vi "S4GUI_002.vi"(7 "Tab ObsEng":enum32{"Obs", "CCD modes", "Eng"}(tab)) -> ()   [LabVIEW 2018] (continued)
                    n514 = Number To Decimal String(number=w1082) -> (decimal integer string=w1084:string)  [unwired: 1 in]
                    n515 = Concatenate Strings("Disk Storage ", w1084, "%" ("string")) -> (w1081:string)
                    n516 = property on="Disk Storage ch3" class="Slide (strict)"("Caption.Text"=w1081) -> ()  [unwired: 2 in, 2 out]
                  }
                  frame #6 {
                    w1110 = cluster{u32, u32}[] [{16711680, 16711680}, {15400704, 15400704}, {16776722, 0}, {16776722, 0}]  # amarelo
                    w1109 = cluster{u32, u32}[] [{16711680, 16711680}, {6618880, 6618880}, {16776722, 0}, {16776722, 0}]  # verde
                    # "Se ocupacao do disco maior que\n90%, barra em vermelho."
                    # "Atualiza status CANAL4"
                    n517 = Unbundle By Name(w1122) -> ("Frames done"=w1117:u32, "connection"=→"Channel 4" →"setupCH4":bool, "conf runing"=w1121:bool, "UsedDisk"=w1103:u16, "operational"=w1107:bool)
                    "Exposures Done ch4" <- w1117
                    "Disk Storage ch4" <- w1103
                    n518 = Number To Decimal String(number=w1117) -> (decimal integer string=w1118:string)  [unwired: 1 in]
                    n519 = Greater?(x=w1103, y=u16 90) -> (0:w1114:bool)
                    n520 = Select(t=u32 16711680, s=w1114, f=u32 16860) -> (s? t:f=w1111:u32)
                    n521 = Concatenate Strings("#Exposures Done ", w1118) -> (w1116:string)
                    n522 = property on="setupCH4" class="Bool (strict)"("Blinking"=w1121) -> ()  [unwired: 2 in, 2 out]
                    n523 = property on="Disk Storage ch4" class="Slide (strict)"("Fill Color"=w1111) -> ()  [unwired: 2 in, 2 out]
                    n524 = Select(t=w1109, s=w1107, f=w1110) -> (s? t:f=w1108:cluster{u32, u32}[])
                    n525 = property on="Exposures Done ch4" class="Slide (strict)"("Caption.Text"=w1116) -> ()  [unwired: 2 in, 2 out]
                    n526 = property on="Channel 4" class="Bool (strict)"("Colors [4]"=w1108) -> ()  [unwired: 2 in, 2 out]
                    n527 = Number To Decimal String(number=w1103) -> (decimal integer string=w1105:string)  [unwired: 1 in]
                    n528 = Concatenate Strings("Disk Storage ", w1105, "%" ("string")) -> (w1102:string)
                    n529 = property on="Disk Storage ch4" class="Slide (strict)"("Caption.Text"=w1102) -> ()  [unwired: 2 in, 2 out]
                  }
                }
              }
              frame #9 {
                n530 = Unbundle By Name(w1128) -> ("Instrument Status.mode"=w1127:bool)
                n531 = case shown="True" w1127 {
                  tunnel: [0 ("t") w1141] -> w1124
                  tunnel: w1128 -> [_ w1130]
                  frame False {
                    # "Fotometria: #PSD = 0"
                  }
                  frame True {
                    # "Polarimetria: calcula #PSD"
                    n532 = Unbundle By Name(w1130) -> ("WPROT seq"=w1134:u16)
                    n533 = Number To Boolean Array(number=w1134) -> (Boolean array=w1133:bool[])
                    n534 = for {
                      shift-right: [w1145] -> w1136
                      shift-left: 0 -> [w1143]
                      tunnel: w1133 -> [w1142] mode=indexing
                      # "calcula qtd de 1s"
                      n535 = Increment(x=w1143) -> (x+1=w1144:i32)
                      n536 = Select(t=w1144, s=w1142, f=w1143) -> (s? t:f=w1145:i32)
                    }
                    n537 = property on="#Pol. Seq. Done" class="Slide (strict)"() -> ("Scale.Maximum"=w1135:dbl)  [unwired: 2 in, 2 out]
                    n538 = To Long Integer(number=w1135) -> (32bit integer=w1137:i32)
                    n539 = Subtract(x=w1137, y=w1136) -> (x-y=w1138:i32)
                    n540 = Decrement(x=w1138) -> (x-1=w1140:i32)
                    n541 = Less Than 0?(x=w1140) -> (x < 0?=w1139:bool)
                    n542 = Select(t=0, s=w1139, f=w1140) -> (s? t:f=w1141:i32)
                  }
                }
                "#Pol. Seq. Done" <- w1124
                n543 = Number To Decimal String(number=w1124) -> (decimal integer string=w1125:string)  [unwired: 1 in]
                n544 = Concatenate Strings("#Pol. Seq. Done ", w1125) -> (w1123:string)
                n545 = property on="#Pol. Seq. Done" class="Slide (strict)"("Caption.Text"=w1123) -> ()  [unwired: 2 in, 2 out]
              }
              frame #10 {
                # "OVJ 2022-12-12: \nA visibilidade do Tab ObsEng sempre \nacompanha a habilitação do tab4."
                n546 = Unbundle By Name(w1155) -> ("Cluster ExpMode.tab4"=w1149:T12, "Cluster Polarimetry"=w1176:T23, "Cluster Mode Sync"=w1183:T24)
                n547 = case shown="\"Enabled\", Default" w1149 {
                  tunnel: [TRUE ("Tabs Visible?") w1185] -> w1154
                  frame "Enabled", Default {
                  }
                  frame "Disabled and Grayed Out" {
                    n548 = disable-structure shown="Enabled" {
                      disable-tunnel: [TRUE ("Tabs Visible?") FALSE ("Tabs Visible?")] -> w1185
                      frame Disabled {
                        # "DEBUG"
                      }
                      frame Enabled {
                      }
                    }
                  }
                }
                n549 = property on="Tab Acq Type" class="TabCtl (strict)"("DisabledEnum"=w1149) -> (error out=w1153:errorcluster)  [unwired: 2 in, 1 out]
                n550 = Unbundle By Name(w1183) -> ("Start SM Text"=w1182:string, "Star SM"=w1151:T12, "Pause SM"=w1181:T12, "Stop SM"=w1180:T12, "Abort SM"=w1179:T12, "#Cycles"=w1178:T12, "SSM"=w1177:T12, "Set SM"=w1146:T12, "#Index Cycles"=w1152:T12)
                n551 = property on="Observer" class="Str"(error in=w1153, "DisabledEnum"=w1149) -> (error out=w1148:errorcluster)  [unwired: 1 in, 1 out]
                n552 = property on="Tab ObsEng" class="TabCtl (strict)"("Tabs Visible?"=w1154) -> ()  [unwired: 2 in, 2 out]
                n553 = property on="Project ID" class="Str"(error in=w1148, "DisabledEnum"=w1149) -> (error out=w1147:errorcluster)  [unwired: 1 in, 1 out]
                n554 = property on="set keywords" class="Bool"(error in=w1147, "DisabledEnum"=w1146) -> (error out=w1150:errorcluster)  [unwired: 1 in, 1 out]
                n555 = property on="Start SM" class="Bool"("BoolText.Text"=w1182) -> ()  [unwired: 2 in, 2 out]
                n556 = property on="#Cycles Done" class="Slide (strict)"("DisabledEnum"=w1152) -> ()  [unwired: 2 in, 2 out]
                n557 = property on="Start SM" class="Bool"("DisabledEnum"=w1151) -> ()  [unwired: 2 in, 2 out]
                n558 = property on="Stop SM" class="Bool"("DisabledEnum"=w1180) -> ()  [unwired: 2 in, 2 out]
                n559 = property on="Abort SM" class="Bool"("DisabledEnum"=w1179) -> ()  [unwired: 2 in, 2 out]
                n560 = property on="Pause SM" class="Bool"("DisabledEnum"=w1181) -> ()  [unwired: 2 in, 2 out]
                n561 = property on="# Cycles" class="DigNum (strict)"("DisabledEnum"=w1178) -> ()  [unwired: 2 in, 2 out]
                n562 = property on="SSM" class="Ring (strict)"("DisabledEnum"=w1177) -> ()  [unwired: 2 in, 2 out]
                n563 = property on="set Observer" class="Bool"(error in=w1150, "DisabledEnum"=w1146) -> ()  [unwired: 1 in, 2 out]
                n564 = Unbundle By Name(w1176) -> ("Lambda Selector"=w1175:T12, "Calibrator Selector"=w1174:T12, "Set Waveplate"=w1173:T12, "Select Positions"=w1172:T12, "P0"=w1171:T12, "P8"=w1170:T12, "P1"=w1169:T12, "P9"=w1168:T12, "P2"=w1167:T12, "P10"=w1166:T12, "P3"=w1165:T12, "P11"=w1164:T12, "P4"=w1163:T12, "P12"=w1162:T12, "P5"=w1161:T12, "P13"=w1160:T12, "P6"=w1159:T12, "P14"=w1158:T12, "P7"=w1157:T12, "P15"=w1156:T12)
                n565 = property on="P0" class="Bool (strict)"("DisabledEnum"=w1171) -> ()  [unwired: 2 in, 2 out]
                n566 = property on="Lambda Selector" class="Ring (strict)"("DisabledEnum"=w1175) -> ()  [unwired: 2 in, 2 out]
                n567 = property on="Calibrator Selector" class="Ring (strict)"("DisabledEnum"=w1174) -> ()  [unwired: 2 in, 2 out]
                n568 = property on="Set Waveplate" class="Bool"("DisabledEnum"=w1173) -> ()  [unwired: 2 in, 2 out]
                n569 = property on="P1" class="Bool (strict)"("DisabledEnum"=w1169) -> ()  [unwired: 2 in, 2 out]
                n570 = property on="P2" class="Bool (strict)"("DisabledEnum"=w1167) -> ()  [unwired: 2 in, 2 out]
                n571 = property on="Select Positions" class="Ring (strict)"("DisabledEnum"=w1172) -> ()  [unwired: 2 in, 2 out]
                n572 = property on="P3" class="Bool (strict)"("DisabledEnum"=w1165) -> ()  [unwired: 2 in, 2 out]
                n573 = property on="P4" class="Bool (strict)"("DisabledEnum"=w1163) -> ()  [unwired: 2 in, 2 out]
                n574 = property on="P5" class="Bool (strict)"("DisabledEnum"=w1161) -> ()  [unwired: 2 in, 2 out]
                n575 = property on="P6" class="Bool (strict)"("DisabledEnum"=w1159) -> ()  [unwired: 2 in, 2 out]
                n576 = property on="P7" class="Bool (strict)"("DisabledEnum"=w1157) -> ()  [unwired: 2 in, 2 out]
                n577 = property on="P8" class="Bool (strict)"("DisabledEnum"=w1170) -> ()  [unwired: 2 in, 2 out]
                n578 = property on="P9" class="Bool (strict)"("DisabledEnum"=w1168) -> ()  [unwired: 2 in, 2 out]
                n579 = property on="P10" class="Bool (strict)"("DisabledEnum"=w1166) -> ()  [unwired: 2 in, 2 out]
                n580 = property on="P11" class="Bool (strict)"("DisabledEnum"=w1164) -> ()  [unwired: 2 in, 2 out]
                n581 = property on="P12" class="Bool (strict)"("DisabledEnum"=w1162) -> ()  [unwired: 2 in, 2 out]
                n582 = property on="P15" class="Bool (strict)"("DisabledEnum"=w1156) -> ()  [unwired: 2 in, 2 out]
                n583 = property on="P13" class="Bool (strict)"("DisabledEnum"=w1160) -> ()  [unwired: 2 in, 2 out]
                n584 = property on="P14" class="Bool (strict)"("DisabledEnum"=w1158) -> ()  [unwired: 2 in, 2 out]
              }
              frame #11 {
                n585 = Unbundle By Name(w1202) -> ("Cluster Mode CH1"=w1190:T25, "Cluster Mode Sync"=w1189:T24)
                n586 = Unbundle By Name(w1190) -> ("Start ch1 Text"=w1201:string, "#cycles ch1"=w1200:T12, "Start ch1"=w1199:T12, "Pause ch1"=w1198:T12, "Abort ch1"=w1197:T12, "Stop ch1"=w1196:T12, "Exptime ch1"=w1195:T12, "Exp ch1"=w1194:T12, "Set Cooler"=w1188:T12, "Set Temp"=w1193:T12)
                n587 = Unbundle By Name(w1189) -> ("#Index Cycles"=w1192:T12)
                n588 = case shown="Default" w1192 {
                  tunnel: [T12."Enabled" ("#Index Cycles") T12."Disabled and Grayed Out" ("#Index Cycles")] -> w1191
                  frame "Disabled and Grayed Out" {
                  }
                  frame Default {
                  }
                }
                n589 = property on="Start ch1" class="Bool"("BoolText.Text"=w1201) -> ()  [unwired: 2 in, 2 out]
                n590 = property on="Abort ch1" class="Bool"("DisabledEnum"=w1197) -> ()  [unwired: 2 in, 2 out]
                n591 = property on="Set Temp 1" class="Bool"("DisabledEnum"=w1193) -> ()  [unwired: 2 in, 2 out]
                n592 = property on="Stop ch1" class="Bool"("DisabledEnum"=w1196) -> ()  [unwired: 2 in, 2 out]
                n593 = property on="#cycles ch1" class="DigNum (strict)"("DisabledEnum"=w1200) -> ()  [unwired: 2 in, 2 out]
                n594 = property on="cooler ON 1" class="Bool (strict)"("DisabledEnum"=w1188) -> ()  [unwired: 2 in, 2 out]
                n595 = property on="cooler OFF 1" class="Bool (strict)"("DisabledEnum"=w1188) -> ()  [unwired: 2 in, 2 out]
                n596 = property on="Exptime ch1" class="DigNum (strict)"("DisabledEnum"=w1195) -> ()  [unwired: 2 in, 2 out]
                n597 = property on="Start ch1" class="Bool"("DisabledEnum"=w1199) -> ()  [unwired: 2 in, 2 out]
                n598 = property on="Exp ch1" class="DigNum (strict)"("DisabledEnum"=w1194) -> ()  [unwired: 2 in, 2 out]
                n599 = property on="Cycles Done ch1" class="Slide (strict)"("DisabledEnum"=w1191) -> ()  [unwired: 2 in, 2 out]
                n600 = property on="Pause ch1" class="Bool"("DisabledEnum"=w1198) -> ()  [unwired: 2 in, 2 out]
              }
              frame #12 {
                n601 = Unbundle By Name(w1219) -> ("Cluster Mode CH2"=w1218:T26, "Cluster Mode Sync"=w1207:T24)
                n602 = Unbundle By Name(w1207) -> ("#Index Cycles"=w1208:T12)
                n603 = Unbundle By Name(w1218) -> ("Start ch2 Text"=w1217:string, "#cycles ch2"=w1216:T12, "Start ch2"=w1215:T12, "Pause ch2"=w1214:T12, "Stop ch2"=w1213:T12, "Abort ch2"=w1212:T12, "Exptime ch2"=w1211:T12, "Exp ch2"=w1210:T12, "Set Cooler"=w1205:T12, "Set Temp"=w1209:T12)
                n604 = case shown="\"Disabled and Grayed Out\"" w1208 {
                  tunnel: [T12."Enabled" ("#Index Cycles") T12."Disabled and Grayed Out" ("#Index Cycles")] -> w1206
                  frame "Disabled and Grayed Out" {
                  }
                  frame Default {
                  }
                }
                n605 = property on="Start ch2" class="Bool"("BoolText.Text"=w1217) -> ()  [unwired: 2 in, 2 out]
                n606 = property on="Stop ch2" class="Bool"("DisabledEnum"=w1213) -> ()  [unwired: 2 in, 2 out]
                n607 = property on="Abort ch2" class="Bool"("DisabledEnum"=w1212) -> ()  [unwired: 2 in, 2 out]
                n608 = property on="#cycles ch2" class="DigNum (strict)"("DisabledEnum"=w1216) -> ()  [unwired: 2 in, 2 out]
                n609 = property on="Set Temp 2" class="Bool"("DisabledEnum"=w1209) -> ()  [unwired: 2 in, 2 out]
                n610 = property on="Exptime ch2" class="DigNum (strict)"("DisabledEnum"=w1211) -> ()  [unwired: 2 in, 2 out]
                n611 = property on="cooler OFF 2" class="Bool (strict)"("DisabledEnum"=w1205) -> ()  [unwired: 2 in, 2 out]
                n612 = property on="cooler ON 2" class="Bool (strict)"("DisabledEnum"=w1205) -> ()  [unwired: 2 in, 2 out]
                n613 = property on="Start ch2" class="Bool"("DisabledEnum"=w1215) -> ()  [unwired: 2 in, 2 out]
                n614 = property on="Cycles Done ch2" class="Slide (strict)"("DisabledEnum"=w1206) -> ()  [unwired: 2 in, 2 out]
                n615 = property on="Exp ch2" class="DigNum (strict)"("DisabledEnum"=w1210) -> ()  [unwired: 2 in, 2 out]
                n616 = property on="Pause ch2" class="Bool"("DisabledEnum"=w1214) -> ()  [unwired: 2 in, 2 out]
              }
              frame #13 {
                n617 = Unbundle By Name(w1236) -> ("Cluster Mode CH3"=w1235:T27, "Cluster Mode Sync"=w1224:T24)
                n618 = Unbundle By Name(w1224) -> ("#Index Cycles"=w1225:T12)
                n619 = Unbundle By Name(w1235) -> ("Start ch3 Text"=w1234:string, "#cycles ch3"=w1233:T12, "Start ch3"=w1232:T12, "Pause ch3"=w1231:T12, "Stop ch3"=w1230:T12, "Abort ch3"=w1229:T12, "Exptime ch3"=w1228:T12, "Exp ch3"=w1227:T12, "Set Cooler"=w1222:T12, "Set Temp"=w1226:T12)
                n620 = case shown="\"Disabled and Grayed Out\"" w1225 {
                  tunnel: [T12."Enabled" ("#Index Cycles") T12."Disabled and Grayed Out" ("#Index Cycles")] -> w1223
                  frame "Disabled and Grayed Out" {
                  }
                  frame Default {
                  }
                }
                n621 = property on="Start ch3" class="Bool"("BoolText.Text"=w1234) -> ()  [unwired: 2 in, 2 out]
                n622 = property on="Stop ch3" class="Bool"("DisabledEnum"=w1230) -> ()  [unwired: 2 in, 2 out]
                n623 = property on="Abort ch3" class="Bool"("DisabledEnum"=w1229) -> ()  [unwired: 2 in, 2 out]
                n624 = property on="Cycles Done ch3" class="Slide (strict)"("DisabledEnum"=w1223) -> ()  [unwired: 2 in, 2 out]
                n625 = property on="#cycles ch3" class="DigNum (strict)"("DisabledEnum"=w1233) -> ()  [unwired: 2 in, 2 out]
                n626 = property on="cooler OFF 3" class="Bool (strict)"("DisabledEnum"=w1222) -> ()  [unwired: 2 in, 2 out]
                n627 = property on="Set Temp 3" class="Bool"("DisabledEnum"=w1226) -> ()  [unwired: 2 in, 2 out]
                n628 = property on="cooler ON 3" class="Bool (strict)"("DisabledEnum"=w1222) -> ()  [unwired: 2 in, 2 out]
                n629 = property on="Exptime ch3" class="DigNum (strict)"("DisabledEnum"=w1228) -> ()  [unwired: 2 in, 2 out]
                n630 = property on="Start ch3" class="Bool"("DisabledEnum"=w1232) -> ()  [unwired: 2 in, 2 out]
                n631 = property on="Exp ch3" class="DigNum (strict)"("DisabledEnum"=w1227) -> ()  [unwired: 2 in, 2 out]
                n632 = property on="Pause ch3" class="Bool"("DisabledEnum"=w1231) -> ()  [unwired: 2 in, 2 out]
              }
              frame #14 {
                n633 = Unbundle By Name(w1253) -> ("Cluster Mode CH4"=w1252:T28, "Cluster Mode Sync"=w1241:T24)
                n634 = Unbundle By Name(w1241) -> ("#Index Cycles"=w1242:T12)
                n635 = Unbundle By Name(w1252) -> ("Start ch4 Text"=w1251:string, "#cycles ch4"=w1250:T12, "Start ch4"=w1249:T12, "Pause ch4"=w1248:T12, "Stop ch4"=w1247:T12, "Abort ch4"=w1246:T12, "Exptime ch4"=w1245:T12, "Exp ch4"=w1244:T12, "Set Cooler"=w1239:T12, "Set Temp"=w1243:T12)
                n636 = case shown="\"Disabled and Grayed Out\"" w1242 {
                  tunnel: [T12."Enabled" ("#Index Cycles") T12."Disabled and Grayed Out" ("#Index Cycles")] -> w1240
                  frame "Disabled and Grayed Out" {
                  }
                  frame Default {
                  }
                }
                n637 = property on="Start ch4" class="Bool"("BoolText.Text"=w1251) -> ()  [unwired: 2 in, 2 out]
                n638 = property on="Stop ch4" class="Bool"("DisabledEnum"=w1247) -> ()  [unwired: 2 in, 2 out]
                n639 = property on="Abort ch4" class="Bool"("DisabledEnum"=w1246) -> ()  [unwired: 2 in, 2 out]
                n640 = property on="#cycles ch4" class="DigNum (strict)"("DisabledEnum"=w1250) -> ()  [unwired: 2 in, 2 out]
                n641 = property on="Set Temp 4" class="Bool"("DisabledEnum"=w1243) -> ()  [unwired: 2 in, 2 out]
                n642 = property on="cooler ON 4" class="Bool (strict)"("DisabledEnum"=w1239) -> ()  [unwired: 2 in, 2 out]
                n643 = property on="cooler OFF 4" class="Bool (strict)"("DisabledEnum"=w1239) -> ()  [unwired: 2 in, 2 out]
                n644 = property on="Exptime ch4" class="DigNum (strict)"("DisabledEnum"=w1245) -> ()  [unwired: 2 in, 2 out]
                n645 = property on="Cycles Done ch4" class="Slide (strict)"("DisabledEnum"=w1240) -> ()  [unwired: 2 in, 2 out]
                n646 = property on="Start ch4" class="Bool"("DisabledEnum"=w1249) -> ()  [unwired: 2 in, 2 out]
                n647 = property on="Exp ch4" class="DigNum (strict)"("DisabledEnum"=w1244) -> ()  [unwired: 2 in, 2 out]
                n648 = property on="Pause ch4" class="Bool"("DisabledEnum"=w1248) -> ()  [unwired: 2 in, 2 out]
              }
              frame #15 {
                # "Carrega coluna do Channel 1"
                # "Aba:  Eng->Camera"
                n649 = Unbundle By Name(w1320) -> ("ChannelA_CCD"=w1265:T29, "CHA_Checked Params"=w1311:T14, "ChannelA_Status.connection"=w1264:bool)
                n650 = Unbundle By Name(w1311) -> ("ACQUISITION_MODE"=w1289:bool, "TRIGGER_MODE"=w1290:bool, "READ_MODE"=w1291:bool, "PREAMP"=w1299:bool, "READOUT_RATE"=w1300:bool, "VERTICAL_SHIFT_SPEED"=w1301:bool, "EM_MODE"=w1302:bool, "EM_GAIN"=w1292:bool, "SHUTTER_MODE"=w1293:bool, "SHUTTER_TTL"=w1294:bool, "SHUTTER_OPENING_TIME"=w1295:bool, "SHUTTER_CLOSING_TIME"=w1296:bool, "VBIN"=w1297:bool, "HBIN"=w1298:bool, "INITIAL_LINE"=w1303:bool, "INITIAL_COLUMN"=w1308:bool, "FINAL_LINE"=w1310:bool, "FINAL_COLUMN"=w1307:bool, "FRAME_TRANSFER"=w1306:bool, "VERTICAL_CLOCK_VOLTAGE"=w1305:bool, "AD_CHANNEL"=w1304:bool)
                n651 = local read "CH1on"() -> (w1257:bool)
                n652 = Unbundle By Name(w1265) -> ("INITIAL_LINE"=w1287:u16, "INITIAL_COLUMN"=w1286:u16, "FINAL_LINE"=w1285:u16, "FINAL_COLUMN"=w1284:u16, "VBIN"=w1283:u16, "HBIN"=w1282:u16, "PREAMP"=w1281:u8, "EM_GAIN"=w1280:u16, "READOUT_RATE"=w1279:u8, "SHUTTER_OPENNING_TIME"=w1278:u16, "SHUTTER_CLOSING_TIME"=w1277:u16, "VERTICAL_SHIFT_SPEED"=w1276:u8, "READ_MODE"=w1275:u8, "VERTICAL_CLOCK_VOLTAGE"=w1274:u8, "AD_CHANNEL"=w1273:u32, "SHUTTER_MODE"=w1272:u8, "SHUTTER_TTL"=w1271:u8, "TRIGGER_MODE"=w1270:u8, "FRAME_TRANSFER"=w1269:bool, "ACQUISITION_MODE"=w1267:u8, "EM_MODE"=w1266:u8)
                n653 = Equal?(x=w1315, y="none") -> (x = y?=w1312:bool)
                n654 = Equal?(x=w1315, y="default.cfg") -> (x = y?=w1313:bool)
                n655 = Or(x=w1313, y=w1312) -> (x .or. y?=w1314:bool)
                n656 = case shown="True" w1314 {
                  tunnel: [T12."Enabled" ("Disabled") T12."Disabled and Grayed Out" ("Disabled")] -> w1317
                  frame False {
                    # "Se Curr Conf File != default.cfg,\nhabilita botão de Salvar."
                  }
                  frame True {
                    # "Não é permitido salvar em \ncima de default.cfg"
                  }
                }
                n657 = case shown="True" w1264 {
                  tunnel: w1265 -> [_ w1373]
                  tunnel: [w1366 w1372] -> w1263
                  tunnel: [w1366 w1371] -> w1262
                  tunnel: [w1366 w1370] -> w1261
                  tunnel: [w1366 w1369] -> w1260
                  tunnel: [w1366 w1368] -> w1259
                  tunnel: [w1366 w1367] -> w1258
                  frame False {
                    w1366 = "" ("RO1")
                  }
                  frame True {
                    n658 = stacked-sequence "Atualizacao dos indicadores inferiores do CANAL A da tela principal" {
                      tunnel: w1373 -> [w1388 w1391 w1396 w1405 w1408 w1412]
                      tunnel: [w1374 _ _ _ _ _] -> w1372
                      tunnel: [_ w1389 _ _ _ _] -> w1371
                      tunnel: [_ _ w1394 _ _ _] -> w1370
                      tunnel: [_ _ _ w1399 _ _] -> w1369
                      tunnel: [_ _ _ _ w1406 _] -> w1368
                      tunnel: [_ _ _ _ _ w1409] -> w1367
                      frame #0 {
                        # "SubImage"
                        n659 = Unbundle By Name(w1388) -> ("INITIAL_LINE"=w1386:u16, "FINAL_LINE"=w1385:u16, "INITIAL_COLUMN"=w1384:u16, "FINAL_COLUMN"=w1383:u16)
                        n660 = Number To Decimal String(number=w1386) -> (decimal integer string=w1382:string)  [unwired: 1 in]
                        n661 = Number To Decimal String(number=w1385) -> (decimal integer string=w1380:string)  [unwired: 1 in]
                        n662 = Number To Decimal String(number=w1384) -> (decimal integer string=w1378:string)  [unwired: 1 in]
                        n663 = Number To Decimal String(number=w1383) -> (decimal integer string=w1376:string)  [unwired: 1 in]
                        n664 = Concatenate Strings("[", w1382, ":", w1380, ",", w1378, ":", w1376, "]") -> (w1374:string)
                      }
                      frame #1 {
                        # "Em Active"
                        n665 = Unbundle By Name(w1391) -> ("EM_MODE"=w1390:u8)
                        n666 = case shown="0, Default" w1390 {
                          tunnel: ["Electron M." ("EmActive1") "Convent." ("EmActive1")] -> w1389
                          frame 0, Default {
                          }
                          frame 1 {
                          }
                        }
                      }
                      frame #2 {
                        # "Pre Amp"
                        n667 = Unbundle By Name(w1396) -> ("PREAMP"=w1395:u8)
                        n668 = case shown="1" w1395 {
                          tunnel: ["Gain 1" ("EmActive1") "Gain 2" ("EmActive1")] -> w1394
                          frame 0, Default {
                          }
                          frame 1 {
                          }
                        }
                      }
                      frame #3 {
                        # "Binning"
                        n669 = Unbundle By Name(w1405) -> ("VBIN"=w1404:u16, "HBIN"=w1403:u16)
                        n670 = Number To Decimal String(number=w1403) -> (decimal integer string=w1400:string)  [unwired: 1 in]
                        n671 = Number To Decimal String(number=w1404) -> (decimal integer string=w1402:string)  [unwired: 1 in]
                        n672 = Concatenate Strings(w1402, "x", w1400) -> (w1399:string)
                      }
                      frame #4 {
                        # "Gain"
                        n673 = Unbundle By Name(w1408) -> ("EM_GAIN"=w1407:u16)
                        n674 = Number To Decimal String(number=w1407) -> (decimal integer string=w1406:string)  [unwired: 1 in]
                      }
                      frame #5 {
                        # "Readout"
                        n675 = Unbundle By Name(w1412) -> ("EM_MODE"=w1411:u8, "READOUT_RATE"=w1410:u8)
                        n676 = case shown="0, Default" w1411 {
                          tunnel: w1410 -> [w1414 w1420]
                          tunnel: [w1413 w1419] -> w1409
                          frame 0, Default {
                            n677 = case shown="0, Default" w1414 {
                              tunnel: ["30 MHz" ("EmActive1") "20 MHz" ("EmActive1") "10 MHz" ("EmActive1") "1 MHz" ("EmActive1")] -> w1413
                              frame 0, Default {
                              }
                              frame 1 {
                              }
                              frame 2 {
                              }
                              frame 3 {
                              }
                            }
                          }
                          frame 1 {
                            n678 = case shown="1" w1420 {
                              tunnel: ["1 MHz" ("EmActive1") "0.1 MHz" ("EmActive1")] -> w1419
                              frame 0, Default {
                              }
                              frame 1 {
                              }
                            }
                          }
                        }
                      }
                    }
                  }
                }
                n679 = case shown="False" w1257 {
                  tunnel: w1310 -> [_ w1365]
                  tunnel: w1308 -> [_ w1361]
                  tunnel: w1307 -> [_ w1359]
                  tunnel: w1306 -> [_ w1355]
                  tunnel: w1305 -> [_ w1354]
                  tunnel: w1304 -> [_ w1353]
                  tunnel: w1303 -> [_ w1345]
                  tunnel: w1302 -> [_ w1337]
                  tunnel: w1301 -> [_ w1336]
                  tunnel: w1300 -> [_ w1335]
                  tunnel: w1299 -> [_ w1334]
                  tunnel: w1298 -> [_ w1333]
                  tunnel: w1297 -> [_ w1332]
                  tunnel: w1296 -> [_ w1331]
                  tunnel: w1295 -> [_ w1330]
                  tunnel: w1294 -> [_ w1329]
                  tunnel: w1293 -> [_ w1328]
                  tunnel: w1292 -> [_ w1327]
                  tunnel: w1291 -> [_ w1326]
                  tunnel: w1290 -> [_ w1325]
                  tunnel: w1289 -> [_ w1324]
                  tunnel: [T12."Disabled and Grayed Out" ("Disabled") T12."Enabled" ("Disabled")] -> w1256
                  frame False {
                    w1321 = FALSE
                    n680 = property on="Image FInal Column" class="DigNum (strict)"("Blinking"=w1321) -> ()  [unwired: 2 in, 2 out]
                    n681 = property on="Frame Transfer" class="Bool (strict)"("Blinking"=w1321) -> ()  [unwired: 2 in, 2 out]
                    n682 = property on="Vertical Clock Voltage" class="Ring (strict)"("Blinking"=w1321) -> ()  [unwired: 2 in, 2 out]
                    n683 = property on="A/D  Channel" class="DigNum (strict)"("Blinking"=w1321) -> ()  [unwired: 2 in, 2 out]
                    n684 = property on="Image Initial Line" class="DigNum (strict)"("Blinking"=w1321) -> ()  [unwired: 2 in, 2 out]
                    n685 = property on="Image Initial Column" class="DigNum (strict)"("Blinking"=w1321) -> ()  [unwired: 2 in, 2 out]
                    n686 = property on="Image Final Line" class="DigNum (strict)"("Blinking"=w1321) -> ()  [unwired: 2 in, 2 out]
                    n687 = property on="Shutter Openning Time" class="DigNum (strict)"("Blinking"=w1321) -> ()  [unwired: 2 in, 2 out]
                    n688 = property on="Shutter Closing Time" class="DigNum (strict)"("Blinking"=w1321) -> ()  [unwired: 2 in, 2 out]
                    n689 = property on="Vertical Binning" class="DigNum (strict)"("Blinking"=w1321) -> ()  [unwired: 2 in, 2 out]
                    n690 = property on="Horizontal Binning" class="DigNum (strict)"("Blinking"=w1321) -> ()  [unwired: 2 in, 2 out]
                    n691 = property on="CCD EM Gain" class="DigNum (strict)"("Blinking"=w1321) -> ()  [unwired: 2 in, 2 out]
                    n692 = property on="Shutter Mode" class="Ring (strict)"("Blinking"=w1321) -> ()  [unwired: 2 in, 2 out]
                    n693 = property on="Shutter TTL" class="Ring (strict)"("Blinking"=w1321) -> ()  [unwired: 2 in, 2 out]
                    n694 = property on="Acquisition Mode" class="Ring (strict)"("Blinking"=w1321) -> ()  [unwired: 2 in, 2 out]
                    n695 = property on="Readout Rate" class="Ring (strict)"("Blinking"=w1321) -> ()  [unwired: 2 in, 2 out]
                    n696 = property on="Vertical Shift Speed" class="Ring (strict)"("Blinking"=w1321) -> ()  [unwired: 2 in, 2 out]
                    n697 = property on="CCD EM Mode" class="Ring (strict)"("Blinking"=w1321) -> ()  [unwired: 2 in, 2 out]
                    n698 = property on="Trigger Mode" class="Ring (strict)"("Blinking"=w1321) -> ()  [unwired: 2 in, 2 out]
                    n699 = property on="Read Mode" class="Ring (strict)"("Blinking"=w1321) -> ()  [unwired: 2 in, 2 out]
                    n700 = property on="Pre-amplification Gain" class="Ring (strict)"("Blinking"=w1321) -> ()  [unwired: 2 in, 2 out]
                  }
                  frame True {
                    n701 = Not(x=w1359) -> (.not. x?=w1360:bool)
                    n702 = Not(x=w1355) -> (.not. x?=w1357:bool)
                    n703 = Not(x=w1354) -> (.not. x?=w1358:bool)
                    n704 = Not(x=w1353) -> (.not. x?=w1356:bool)
                    n705 = Not(x=w1345) -> (.not. x?=w1363:bool)
                    n706 = Not(x=w1361) -> (.not. x?=w1362:bool)
                    n707 = Not(x=w1365) -> (.not. x?=w1364:bool)
                    n708 = property on="Image FInal Column" class="DigNum (strict)"("Blinking"=w1360) -> ()  [unwired: 2 in, 2 out]
                    n709 = property on="Frame Transfer" class="Bool (strict)"("Blinking"=w1357) -> ()  [unwired: 2 in, 2 out]
                    n710 = property on="Vertical Clock Voltage" class="Ring (strict)"("Blinking"=w1358) -> ()  [unwired: 2 in, 2 out]
                    n711 = property on="A/D  Channel" class="DigNum (strict)"("Blinking"=w1356) -> ()  [unwired: 2 in, 2 out]
                    n712 = property on="Image Initial Line" class="DigNum (strict)"("Blinking"=w1363) -> ()  [unwired: 2 in, 2 out]
                    n713 = property on="Image Initial Column" class="DigNum (strict)"("Blinking"=w1362) -> ()  [unwired: 2 in, 2 out]
                    n714 = property on="Image Final Line" class="DigNum (strict)"("Blinking"=w1364) -> ()  [unwired: 2 in, 2 out]
                    n715 = Not(x=w1330) -> (.not. x?=w1349:bool)
                    n716 = Not(x=w1331) -> (.not. x?=w1351:bool)
                    n717 = Not(x=w1332) -> (.not. x?=w1350:bool)
                    n718 = Not(x=w1333) -> (.not. x?=w1352:bool)
                    n719 = Not(x=w1327) -> (.not. x?=w1347:bool)
                    n720 = Not(x=w1328) -> (.not. x?=w1348:bool)
                    n721 = Not(x=w1329) -> (.not. x?=w1346:bool)
                    n722 = property on="Shutter Openning Time" class="DigNum (strict)"("Blinking"=w1349) -> ()  [unwired: 2 in, 2 out]
                    n723 = property on="Shutter Closing Time" class="DigNum (strict)"("Blinking"=w1351) -> ()  [unwired: 2 in, 2 out]
                    n724 = property on="Vertical Binning" class="DigNum (strict)"("Blinking"=w1350) -> ()  [unwired: 2 in, 2 out]
                    n725 = property on="Horizontal Binning" class="DigNum (strict)"("Blinking"=w1352) -> ()  [unwired: 2 in, 2 out]
                    n726 = property on="CCD EM Gain" class="DigNum (strict)"("Blinking"=w1347) -> ()  [unwired: 2 in, 2 out]
                    n727 = property on="Shutter Mode" class="Ring (strict)"("Blinking"=w1348) -> ()  [unwired: 2 in, 2 out]
                    n728 = property on="Shutter TTL" class="Ring (strict)"("Blinking"=w1346) -> ()  [unwired: 2 in, 2 out]
                    n729 = Not(x=w1324) -> (.not. x?=w1338:bool)
                    n730 = Not(x=w1335) -> (.not. x?=w1341:bool)
                    n731 = Not(x=w1336) -> (.not. x?=w1339:bool)
                    n732 = Not(x=w1337) -> (.not. x?=w1340:bool)
                    n733 = Not(x=w1325) -> (.not. x?=w1343:bool)
                    n734 = Not(x=w1326) -> (.not. x?=w1342:bool)
                    n735 = Not(x=w1334) -> (.not. x?=w1344:bool)
                    n736 = property on="Acquisition Mode" class="Ring (strict)"("Blinking"=w1338) -> ()  [unwired: 2 in, 2 out]
                    n737 = property on="Readout Rate" class="Ring (strict)"("Blinking"=w1341) -> ()  [unwired: 2 in, 2 out]
                    n738 = property on="Vertical Shift Speed" class="Ring (strict)"("Blinking"=w1339) -> ()  [unwired: 2 in, 2 out]
                    n739 = property on="CCD EM Mode" class="Ring (strict)"("Blinking"=w1340) -> ()  [unwired: 2 in, 2 out]
                    n740 = property on="Trigger Mode" class="Ring (strict)"("Blinking"=w1343) -> ()  [unwired: 2 in, 2 out]
                    n741 = property on="Read Mode" class="Ring (strict)"("Blinking"=w1342) -> ()  [unwired: 2 in, 2 out]
                    n742 = property on="Pre-amplification Gain" class="Ring (strict)"("Blinking"=w1344) -> ()  [unwired: 2 in, 2 out]
                  }
                }
                n743 = property on="Save Button" class="Bool (strict)"("DisabledEnum"=w1317) -> ()  [unwired: 2 in, 2 out]
                n744 = First Call?() -> (First Call?: T/F=w1288:bool)
                n745 = case shown="True" w1288 {
                  tunnel: w1287 -> [_ w1443]
                  tunnel: w1286 -> [_ w1442]
                  tunnel: w1285 -> [_ w1441]
                  tunnel: w1284 -> [_ w1440]
                  tunnel: w1283 -> [_ w1439]
                  tunnel: w1282 -> [_ w1438]
                  tunnel: w1281 -> [_ w1437]
                  tunnel: w1280 -> [_ w1436]
                  tunnel: w1279 -> [_ w1435]
                  tunnel: w1278 -> [_ w1434]
                  tunnel: w1277 -> [_ w1433]
                  tunnel: w1276 -> [_ w1432]
                  tunnel: w1275 -> [_ w1431]
                  tunnel: w1274 -> [_ w1430]
                  tunnel: w1273 -> [_ w1429]
                  tunnel: w1272 -> [_ w1428]
                  tunnel: w1271 -> [_ w1427]
                  tunnel: w1270 -> [_ w1426]
                  tunnel: w1269 -> [_ w1425]
                  tunnel: w1267 -> [_ w1424]
                  tunnel: w1266 -> [_ w1423]
                  frame False {
                  }
                  frame True {
                    n746 = local read "Input Cluster"() -> (w1447:T8)
                    n747 = Unbundle By Name(w1447) -> ("Parameters"=w1445:T5)
                    n748 = Bundle By Name(cluster=w1445, "Image \nInitial Line"=w1443, "Image\nInitial Column"=w1442, "Image\nFinal Line"=w1441, "Image\nFInal Column"=w1440, "Vertical\nBinning"=w1439, "Horizontal\nBinning"=w1438, "Pre-amplification\nGain"=w1437, "CCD\nEM Gain"=w1436, "Readout\nRate"=w1435, "Shutter\nOpenning Time"=w1434, "Shutter\nClosing Time"=w1433, "Vertical\nShift Speed"=w1432, "Read\nMode"=w1431, "Vertical\nClock Voltage"=w1430, "A/D \nChannel"=w1429, "Shutter\nMode"=w1428, "Shutter\nTTL"=w1427, "Trigger\nMode"=w1426, "Frame\nTransfer"=w1425, "Acquisition\nMode"=w1424, "CCD \nEM Mode"=w1423) -> (w1444:T5)
                    n749 = Bundle By Name(cluster=w1447, "Parameters"=w1444) -> (w1446:T8)
                    n750 = local write "Input Cluster"(w1446) -> ()
                  }
                }
                n751 = local read "Cameras Cluster"() -> (w1319:T7)
                n752 = Bundle By Name(cluster=w1319, "Current Configuration.Image Initial Line"=w1287, "Current Configuration.Image Initial Column"=w1286, "Current Configuration.Image Final Line"=w1285, "Current Configuration.Image FInal Column"=w1284, "Current Configuration.Vertical Binning"=w1283, "Current Configuration.Horizontal Binning"=w1282, "Current Configuration.Pre-amplification Gain"=w1281, "Current Configuration.CCD EM Gain"=w1280, "Current Configuration.Readout Rate"=w1279, "Current Configuration.Shutter Openning Time"=w1278, "Current Configuration.Shutter Closing Time"=w1277, "Current Configuration.Vertical Shift Speed"=w1276, "Current Configuration.Read Mode"=w1275, "Current Configuration.Vertical Clock Voltage"=w1274, "Current Configuration.A/D  Channel"=w1273, "Current Configuration.Shutter Mode"=w1272, "Current Configuration.Shutter TTL"=w1271, "Current Configuration.Trigger Mode"=w1270, "Current Configuration.Frame Transfer"=w1269, "Current Configuration.Acquisition Mode"=w1267, "Current Configuration.CCD EM Mode"=w1266) -> (w1268:T7)
                n753 = local write "RO1"(w1258) -> ()
                n754 = local write "SI1"(w1263) -> ()
                n755 = local write "EA1"(w1262) -> ()
                n756 = local write "PA1"(w1261) -> ()
                n757 = local write "B1"(w1260) -> ()
                n758 = local write "G1"(w1259) -> ()
                n759 = local write "Cameras Cluster"(w1268) -> ()
                n760 = Compound Arithmetic op=AND(w1289, w1290, w1291, w1299, w1300, w1301, w1302, w1292, w1293, w1294, w1295, w1296, w1297, w1298, w1303, w1308, w1310, w1307, w1306, w1305, w1304) -> (→"CCD checked 1":bool)
                n761 = property on="Shutter Openning Time" class="DigNum (strict)"("DisabledEnum"=w1256) -> ()  [unwired: 2 in, 2 out]
                n762 = property on="Shutter Closing Time" class="DigNum (strict)"("DisabledEnum"=w1256) -> ()  [unwired: 2 in, 2 out]
                n763 = property on="Vertical Binning" class="DigNum (strict)"("DisabledEnum"=w1256) -> ()  [unwired: 2 in, 2 out]
                n764 = property on="Horizontal Binning" class="DigNum (strict)"("DisabledEnum"=w1256) -> ()  [unwired: 2 in, 2 out]
                n765 = property on="CCD EM Gain" class="DigNum (strict)"("DisabledEnum"=w1256) -> ()  [unwired: 2 in, 2 out]
                n766 = property on="Shutter Mode" class="Ring (strict)"("DisabledEnum"=w1256) -> ()  [unwired: 2 in, 2 out]
                n767 = property on="Shutter TTL" class="Ring (strict)"("DisabledEnum"=w1256) -> ()  [unwired: 2 in, 2 out]
                n768 = property on="Acquisition Mode" class="Ring (strict)"("DisabledEnum"=w1256) -> ()  [unwired: 2 in, 2 out]
                n769 = property on="Readout Rate" class="Ring (strict)"("DisabledEnum"=w1256) -> ()  [unwired: 2 in, 2 out]
                n770 = property on="Vertical Shift Speed" class="Ring (strict)"("DisabledEnum"=w1256) -> ()  [unwired: 2 in, 2 out]
                n771 = property on="CCD EM Mode" class="Ring (strict)"("DisabledEnum"=w1256) -> ()  [unwired: 2 in, 2 out]
                n772 = property on="Trigger Mode" class="Ring (strict)"("DisabledEnum"=w1256) -> ()  [unwired: 2 in, 2 out]
                n773 = property on="Read Mode" class="Ring (strict)"("DisabledEnum"=w1256) -> ()  [unwired: 2 in, 2 out]
                n774 = property on="Pre-amplification Gain" class="Ring (strict)"("DisabledEnum"=w1256) -> ()  [unwired: 2 in, 2 out]
                n775 = property on="Image FInal Column" class="DigNum (strict)"("DisabledEnum"=w1256) -> ()  [unwired: 2 in, 2 out]
                n776 = property on="Frame Transfer" class="Bool (strict)"("DisabledEnum"=w1256) -> ()  [unwired: 2 in, 2 out]
                n777 = property on="Vertical Clock Voltage" class="Ring (strict)"("DisabledEnum"=w1256) -> ()  [unwired: 2 in, 2 out]
                n778 = property on="A/D  Channel" class="DigNum (strict)"("DisabledEnum"=w1256) -> ()  [unwired: 2 in, 2 out]
                n779 = property on="Image Initial Line" class="DigNum (strict)"("DisabledEnum"=w1256) -> ()  [unwired: 2 in, 2 out]
                n780 = property on="Image Initial Column" class="DigNum (strict)"("DisabledEnum"=w1256) -> ()  [unwired: 2 in, 2 out]
                n781 = property on="Image Final Line" class="DigNum (strict)"("DisabledEnum"=w1256) -> ()  [unwired: 2 in, 2 out]
                "Current Configuration File:" <- w1315
              }
              frame #16 {
                # "Carrega coluna do Channel 2"
                # "Aba:  Eng->Camera"
                n782 = Unbundle By Name(w1506) -> ("ChannelB_CCD"=w1462:T29, "CHB_Checked Params"=w1463:T14, "ChannelB_Status.connection"=w1461:bool)
                n783 = Unbundle By Name(w1463) -> ("ACQUISITION_MODE"=w1479:bool, "TRIGGER_MODE"=w1478:bool, "READ_MODE"=w1477:bool, "PREAMP"=w1476:bool, "READOUT_RATE"=w1452:bool, "VERTICAL_SHIFT_SPEED"=w1451:bool, "EM_MODE"=w1475:bool, "EM_GAIN"=w1486:bool, "SHUTTER_MODE"=w1485:bool, "SHUTTER_TTL"=w1484:bool, "SHUTTER_OPENING_TIME"=w1483:bool, "SHUTTER_CLOSING_TIME"=w1482:bool, "VBIN"=w1481:bool, "HBIN"=w1480:bool, "INITIAL_LINE"=w1493:bool, "INITIAL_COLUMN"=w1492:bool, "FINAL_LINE"=w1491:bool, "FINAL_COLUMN"=w1490:bool, "FRAME_TRANSFER"=w1489:bool, "VERTICAL_CLOCK_VOLTAGE"=w1488:bool, "AD_CHANNEL"=w1487:bool)
                n784 = case shown="True" w1461 {
                  tunnel: w1462 -> [_ w1563]
                  tunnel: [w1556 w1562] -> w1460
                  tunnel: [w1556 w1561] -> w1459
                  tunnel: [w1556 w1560] -> w1458
                  tunnel: [w1556 w1559] -> w1457
                  tunnel: [w1556 w1558] -> w1456
                  tunnel: [w1556 w1557] -> w1455
                  frame False {
                    w1556 = "" ("EmActive1")
                  }
                  frame True {
                    n785 = stacked-sequence "Atualizacao dos indicadores inferiores do CANAL B da tela principal" {
                      tunnel: w1563 -> [w1578 w1581 w1586 w1595 w1598 w1602]
                      tunnel: [_ w1579 _ _ _ _] -> w1562
                      tunnel: [_ _ w1584 _ _ _] -> w1561
                      tunnel: [_ _ _ w1589 _ _] -> w1560
                      tunnel: [_ _ _ _ w1596 _] -> w1559
                      tunnel: [_ _ _ _ _ w1599] -> w1558
                      tunnel: [w1564 _ _ _ _ _] -> w1557
                      frame #0 {
                        # "SubImage"
                        n786 = Unbundle By Name(w1578) -> ("INITIAL_LINE"=w1576:u16, "FINAL_LINE"=w1575:u16, "INITIAL_COLUMN"=w1574:u16, "FINAL_COLUMN"=w1573:u16)
                        n787 = Number To Decimal String(number=w1576) -> (decimal integer string=w1572:string)  [unwired: 1 in]
                        n788 = Number To Decimal String(number=w1575) -> (decimal integer string=w1570:string)  [unwired: 1 in]
                        n789 = Number To Decimal String(number=w1574) -> (decimal integer string=w1568:string)  [unwired: 1 in]
                        n790 = Number To Decimal String(number=w1573) -> (decimal integer string=w1566:string)  [unwired: 1 in]
                        n791 = Concatenate Strings("[", w1572, ":", w1570, ",", w1568, ":", w1566, "]") -> (w1564:string)
                      }
                      frame #1 {
                        # "Em Active"
                        n792 = Unbundle By Name(w1581) -> ("EM_MODE"=w1580:u8)
                        n793 = case shown="0, Default" w1580 {
                          tunnel: ["Electron M." ("EmActive1") "Convent." ("EmActive1")] -> w1579
                          frame 0, Default {
                          }
                          frame 1 {
                          }
                        }
                      }
                      frame #2 {
                        # "Pre Amp"
                        n794 = Unbundle By Name(w1586) -> ("PREAMP"=w1585:u8)
                        n795 = case shown="1" w1585 {
                          tunnel: ["Gain 1" ("EmActive1") "Gain 2" ("EmActive1")] -> w1584
                          frame 0, Default {
                          }
                          frame 1 {
                          }
                        }
                      }
                      frame #3 {
                        # "Binning"
                        n796 = Unbundle By Name(w1595) -> ("VBIN"=w1594:u16, "HBIN"=w1593:u16)
                        n797 = Number To Decimal String(number=w1593) -> (decimal integer string=w1591:string)  [unwired: 1 in]
                        n798 = Number To Decimal String(number=w1594) -> (decimal integer string=w1592:string)  [unwired: 1 in]
                        n799 = Concatenate Strings(w1592, "x", w1591) -> (w1589:string)
                      }
                      frame #4 {
                        # "Gain"
                        n800 = Unbundle By Name(w1598) -> ("EM_GAIN"=w1597:u16)
                        n801 = Number To Decimal String(number=w1597) -> (decimal integer string=w1596:string)  [unwired: 1 in]
                      }
                      frame #5 {
                        # "Readout"
                        n802 = Unbundle By Name(w1602) -> ("EM_MODE"=w1601:u8, "READOUT_RATE"=w1600:u8)
                        n803 = case shown="0, Default" w1601 {
                          tunnel: w1600 -> [w1604 w1610]
                          tunnel: [w1603 w1609] -> w1599
                          frame 0, Default {
                            n804 = case shown="3" w1604 {
                              tunnel: ["30 MHz" ("EmActive1") "20 MHz" ("EmActive1") "10 MHz" ("EmActive1") "1 MHz" ("EmActive1")] -> w1603
                              frame 0, Default {
                              }
                              frame 1 {
                              }
                              frame 2 {
                              }
                              frame 3 {
                              }
                            }
                          }
                          frame 1 {
                            n805 = case shown="1" w1610 {
                              tunnel: ["1 MHz" ("EmActive1") "0.1 MHz" ("EmActive1")] -> w1609
                              frame 0, Default {
                              }
                              frame 1 {
                              }
                            }
                          }
                        }
                      }
                    }
                  }
                }
                n806 = Unbundle By Name(w1462) -> ("INITIAL_LINE"=w1468:u16, "INITIAL_COLUMN"=w1466:u16, "FINAL_LINE"=w1469:u16, "FINAL_COLUMN"=w1467:u16, "VBIN"=w1472:u16, "HBIN"=w1503:u16, "PREAMP"=w1471:u8, "EM_GAIN"=w1470:u16, "READOUT_RATE"=w1465:u8, "SHUTTER_OPENNING_TIME"=w1502:u16, "SHUTTER_CLOSING_TIME"=w1501:u16, "VERTICAL_SHIFT_SPEED"=w1500:u8, "READ_MODE"=w1499:u8, "VERTICAL_CLOCK_VOLTAGE"=w1498:u8, "AD_CHANNEL"=w1497:u32, "SHUTTER_MODE"=w1494:u8, "SHUTTER_TTL"=w1495:u8, "TRIGGER_MODE"=w1473:u8, "FRAME_TRANSFER"=w1474:bool, "ACQUISITION_MODE"=w1496:u8, "EM_MODE"=w1464:u8)
                n807 = local read "CH2on"() -> (w1454:bool)
                n808 = case shown="False" w1454 {
                  tunnel: w1493 -> [_ w1534]
                  tunnel: w1492 -> [_ w1533]
                  tunnel: w1491 -> [_ w1532]
                  tunnel: w1490 -> [_ w1531]
                  tunnel: w1489 -> [_ w1530]
                  tunnel: w1488 -> [_ w1529]
                  tunnel: w1487 -> [_ w1528]
                  tunnel: w1486 -> [_ w1527]
                  tunnel: w1485 -> [_ w1526]
                  tunnel: w1484 -> [_ w1525]
                  tunnel: w1483 -> [_ w1524]
                  tunnel: w1482 -> [_ w1523]
                  tunnel: w1481 -> [_ w1522]
                  tunnel: w1480 -> [_ w1521]
                  tunnel: w1479 -> [_ w1520]
                  tunnel: w1478 -> [_ w1519]
                  tunnel: w1477 -> [_ w1518]
                  tunnel: w1476 -> [_ w1517]
                  tunnel: w1452 -> [_ w1516]
                  tunnel: w1451 -> [_ w1515]
                  tunnel: w1475 -> [_ w1514]
                  tunnel: [T12."Disabled and Grayed Out" ("Disabled") T12."Enabled" ("Disabled")] -> w1453
                  frame False {
                    w1512 = FALSE ("Blinking")
                    n809 = property on="Image FInal Column 2" class="DigNum (strict)"("Blinking"=w1512) -> ()  [unwired: 2 in, 2 out]
                    n810 = property on="Frame Transfer 2" class="Bool (strict)"("Blinking"=w1512) -> ()  [unwired: 2 in, 2 out]
                    n811 = property on="Vertical Clock Voltage 2" class="Ring (strict)"("Blinking"=w1512) -> ()  [unwired: 2 in, 2 out]
                    n812 = property on="A/D Channel 2" class="DigNum (strict)"("Blinking"=w1512) -> ()  [unwired: 2 in, 2 out]
                    n813 = property on="Image Initial Line 2" class="DigNum (strict)"("Blinking"=w1512) -> ()  [unwired: 2 in, 2 out]
                    n814 = property on="Image Initial Column 2" class="DigNum (strict)"("Blinking"=w1512) -> ()  [unwired: 2 in, 2 out]
                    n815 = property on="Image Final Line 2" class="DigNum (strict)"("Blinking"=w1512) -> ()  [unwired: 2 in, 2 out]
                    n816 = property on="Shutter Openning Time 2" class="DigNum (strict)"("Blinking"=w1512) -> ()  [unwired: 2 in, 2 out]
                    n817 = property on="Shutter Closing Time 2" class="DigNum (strict)"("Blinking"=w1512) -> ()  [unwired: 2 in, 2 out]
                    n818 = property on="Vertical Binning 2" class="DigNum (strict)"("Blinking"=w1512) -> ()  [unwired: 2 in, 2 out]
                    n819 = property on="Horizontal Binning 2" class="DigNum (strict)"("Blinking"=w1512) -> ()  [unwired: 2 in, 2 out]
                    n820 = property on="CCD EM Gain 2" class="DigNum (strict)"("Blinking"=w1512) -> ()  [unwired: 2 in, 2 out]
                    n821 = property on="Shutter Mode 2" class="Ring (strict)"("Blinking"=w1512) -> ()  [unwired: 2 in, 2 out]
                    n822 = property on="Shutter TTL 2" class="Ring (strict)"("Blinking"=w1512) -> ()  [unwired: 2 in, 2 out]
                    n823 = property on="Acquisition Mode 2" class="Ring (strict)"("Blinking"=w1512) -> ()  [unwired: 2 in, 2 out]
                    n824 = property on="Readout Rate 2" class="Ring (strict)"("Blinking"=w1512) -> ()  [unwired: 2 in, 2 out]
                    n825 = property on="Vertical Shift Speed 2" class="Ring (strict)"("Blinking"=w1512) -> ()  [unwired: 2 in, 2 out]
                    n826 = property on="CCD EM Mode 2" class="Ring (strict)"("Blinking"=w1512) -> ()  [unwired: 2 in, 2 out]
                    n827 = property on="Trigger Mode 2" class="Ring (strict)"("Blinking"=w1512) -> ()  [unwired: 2 in, 2 out]
                    n828 = property on="Read Mode 2" class="Ring (strict)"("Blinking"=w1512) -> ()  [unwired: 2 in, 2 out]
                    n829 = property on="Pre-amplification Gain 2" class="Ring (strict)"("Blinking"=w1512) -> ()  [unwired: 2 in, 2 out]
                  }
                  frame True {
                    n830 = Not(x=w1531) -> (.not. x?=w1552:bool)
                    n831 = Not(x=w1530) -> (.not. x?=w1550:bool)
                    n832 = Not(x=w1529) -> (.not. x?=w1551:bool)
                    n833 = Not(x=w1528) -> (.not. x?=w1549:bool)
